vi "isConfigured.vi"(8 "error in (no error)":errorcluster, 11 "ExperimentControl in":refnum<class "ExperimentControl.lvclass">) -> (0 "error out":errorcluster, 2 "configured":bool, 3 "ExperimentControl out":refnum<class "ExperimentControl.lvclass">)   [LabVIEW 2009, in "Views.lvlib" / "ExperimentControl.lvlib" / "ExperimentControl.lvclass"]
uses:
  ExperimentControl.lvclass
  Hal/HWController/HWControllerEvents/HWControllerEvents.lvclass
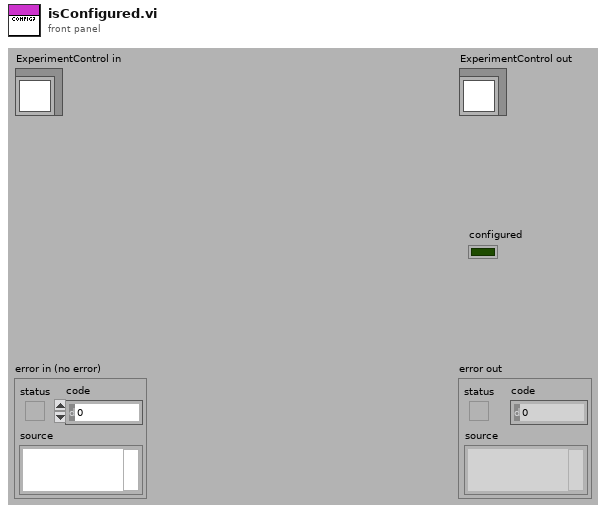
[diagram p1: front panel]
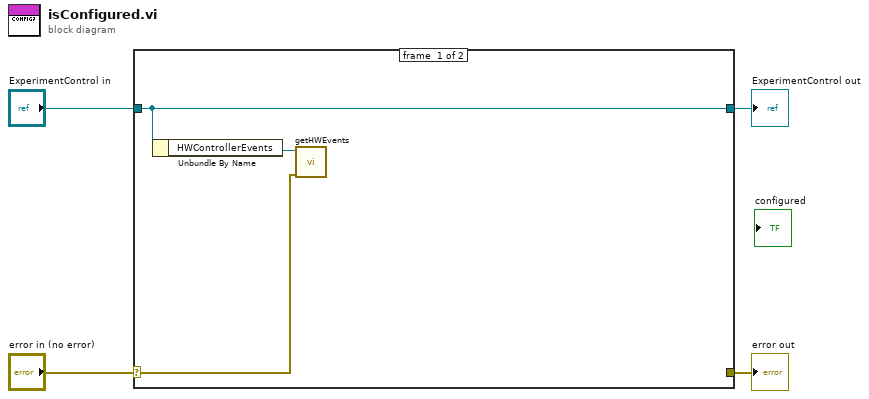
[diagram p0: block diagram]
diagram:
  n1 = case shown="No Error" "error in (no error)" {
    selector: "error in (no error)" -> [w5 w9]
    tunnel: [_ w9] -> w3
    tunnel: [w7 w8] -> w1
    tunnel: "ExperimentControl in" -> [w7 w8]
    frame #0 {
      n2 = Unbundle By Name(w7) -> ("HWControllerEvents"=w6:refnum<class "HWControllerEvents.lvclass">)
      n3 = call-dynamic "getHWEvents.vi"("error in (no error)"=w5, "HWControllerEvents in"=w6) -> ()  [unwired: 6 in, 4 out]
    }
    frame #1 {
    }
  }
  "error out" <- w3
  "ExperimentControl out" <- w1
